vi "synnax channel retrieve keys Single.vi"(0 "Synnax Client in":refnum<class "Synnax Client.lvclass">, 5 "name":string, 11 "error in (no error)":errorcluster) -> (4 "Synnax Client out":refnum<class "Synnax Client.lvclass">, 6 "key":u32, 15 "error out":errorcluster)   [LabVIEW 2026, in "synnax_clib.lvlib" / "Synnax Client.lvclass"]
doc: "SYNNAX_EXPORT int32_t synnax_channel_retrieve_keys(\n SynnaxClient client,\n const char **names,\n uint64_t name_count,\n uint32_t *out_keys,\n SynnaxError err\n);"
uses:
  Synnax Client.lvclass
  Synnax Client.lvclass/Synnax Client.ctl
  synnax_clib.lvlib
  synnax_clib.dll
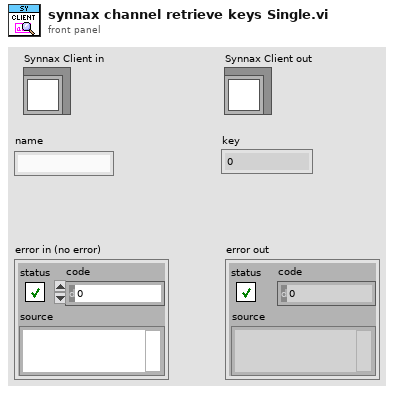
[diagram p1: front panel]
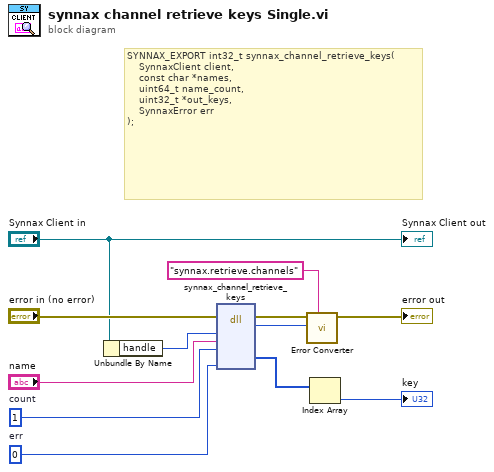
[diagram p0: block diagram]
diagram:
  w4 = u64 1  # count
  w7 = u64 0  # err
  # "SYNNAX_EXPORT int32_t synnax_channel_retrieve_keys(\n    SynnaxClient client,\n    const char *names,\n    uint64_t name_count,\n    uint32_t *out_keys,\n    SynnaxError err\n);"
  n1 = Unbundle By Name("Synnax Client in") -> ("handle"=w2:u64)
  n2 = dll-call lib="C/synnax/client/labview/synnax_clib.*" fn="synnax_channel_retrieve_keys"(error in="error in (no error)", "client"=w2, "names"="name", "name_count"=w4, "err"=w7) -> (error out=w9:errorcluster, "return type"=w11:i32, "out_keys"=w6:u32[])  [unwired: 7 in, 1 out]
  n3 = call "Error Converter.vi"("source"="synnax.retrieve.channels", "error code"=w11, "error in (no error)"=w9) -> ("error out"=→"error out":errorcluster)  [unwired: 8 in]
  n4 = Index Array(array=w6) -> (element=→"key":u32)  [unwired: 1 in]
  "Synnax Client out" <- "Synnax Client in"
